vi "GetGrabberPosition.vi"(8 "error in (no error)":errorcluster, 11 "JKI.Robot.SMO":refnum<class "JKI.Robot.SMO.lvclass">) -> (0 "error out":errorcluster, 2 "SetGrabberPosition":dbl, 3 "JKI.Robot.SMO out":refnum<class "JKI.Robot.SMO.lvclass">)   [LabVIEW 2015, in "JKI.Robot.SMO.lvclass"]
doc: "---------------------------------------------------------------\nJKI State Machine Objects™\nhttp://jki.net/state-machine-objects/\nCopyright (C) 2005-2015, JKI <info@jki.net>\nALL RIGHTS RESERVEDJKI State Machine Objects (SMO) 1.0.0.4\nJKI - JKI\nCopyright (c) 2015, JKI"
uses:
  JKI.Robot.SMO.lvclass
  JKI.Robot.SMO.lvclass/JKI.Robot.SMO.ctl
panel:
  # "For instructions on how to use the JKI State Machine Objects, examples and video tutorials, visit:\nhttp://jki.net/state-machine-objects/\n\nJKI State Machine Objects™\nhttp://jki.net/state-machine-objects/\nCopyright (C) 2005-2015, JKI <info@jki.net>\nALL RIGHTS RESERVED"
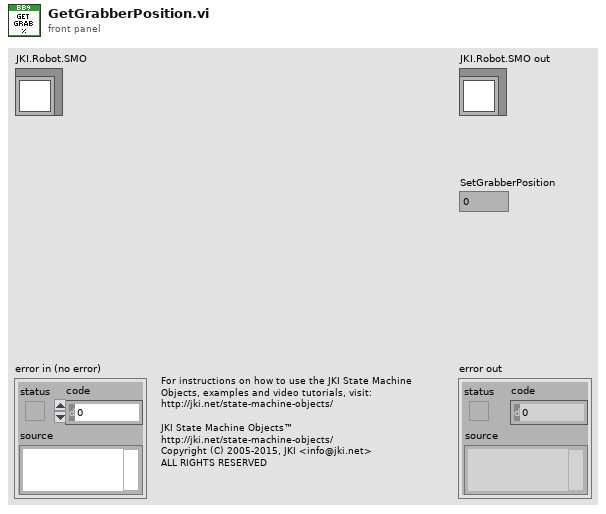
[diagram p1: front panel]
types:
  T1 = typedef "JKI.Robot.SMO.lvclass/PrivateData--Ref.ctl" = refnum<data-value>
  T2 = typedef "JKI.Robot.SMO.lvclass/PrivateData--Cluster.ctl" = cluster{"Configuration":T3, "Public Events":T4, "Robot Position":T5, "Private Events":T6}
  T3 = typedef "JKI.Robot.SMO.lvclass/Configuration--Cluster.ctl" = cluster{"Suffix":string}
  T4 = typedef "JKI.Robot.SMO.lvclass/PublicEvents--Cluster.ctl" = cluster{"Data Changed":refnum<user-event>}
  T5 = typedef "RobotPosition--Cluster.ctl" = cluster{"Claw":dbl, "JointA":dbl, "JointB":dbl, "JointC":dbl, "JointD":dbl}
  T6 = typedef "JKI.Robot.SMO.lvclass/PrivateEvents--Cluster.ctl" = cluster{"SetGrabberPosition":refnum<user-event>, "SetJointRotation":refnum<user-event>}
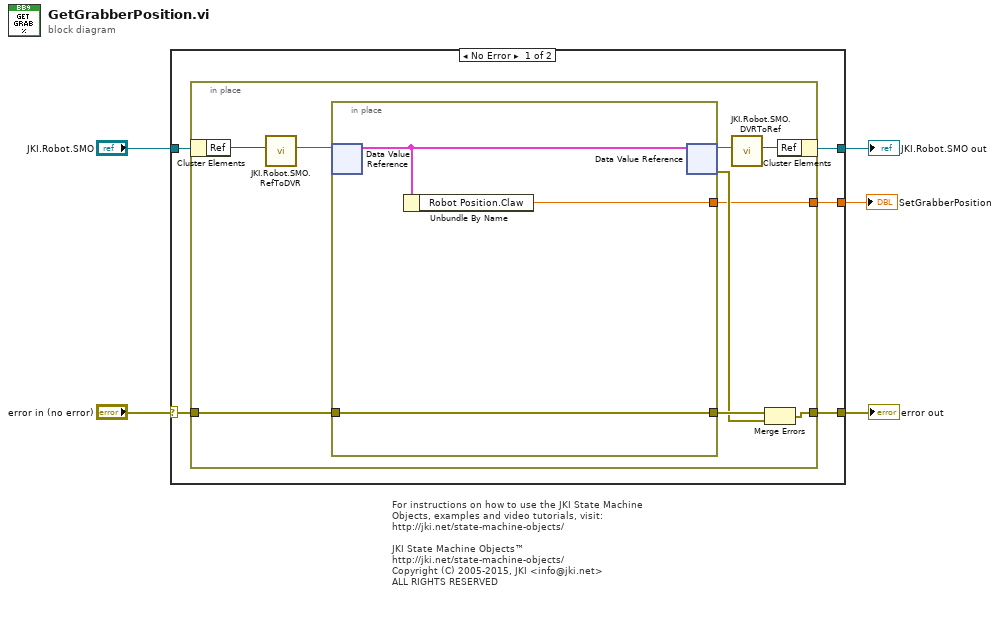
[diagram p0: block diagram]
diagram:
  # "For instructions on how to use the JKI State Machine Objects, examples and video tutorials, visit:\nhttp://jki.net/state-machine-objects/\n\nJKI State Machine Objects™\nhttp://jki.net/state-machine-objects/\nCopyright (C) 2005-2015, JKI <info@jki.net>\nALL RIGHTS RESERVED"
  n1 = case shown="No Error" "error in (no error)" {
    selector: "error in (no error)" -> [w8 w24]
    tunnel: [w7 w24] -> w4
    tunnel: [w9 w23] -> w5
    tunnel: "JKI.Robot.SMO" -> [w10 w23]
    tunnel: [w6 _] -> w1
    frame No Error {
      n2 = in-place {
        in-place-border: w8 -> [w19]
        in-place-border: [w16] -> w7
        in-place-border: [w11] -> w6
        n3 = in-place-cluster #1(w10) -> ("Ref"=w15:u32)
        n4 = call "JKI.Robot.SMO.RefToDVR.vi"("Ref"=w15) -> ("Ref"=w13:T1)  [unwired: 10 in]
        n5 = in-place {
          in-place-border: w19 -> [w20]
          in-place-border: [w20] -> w18
          in-place-border: [w21] -> w11
          n6 = in-place-dvr #2(w13) -> (w22:T2)  [unwired: 1 out]
          n7 = Unbundle By Name(w22) -> ("Robot Position.Claw"=w21:dbl)
          n8 = in-place-dvr #2(w22) -> (w14:T1, w17:errorcluster)
        }
        n9 = call "JKI.Robot.SMO.DVRToRef.vi"("Ref"=w14) -> ("Ref"=w12:u32)  [unwired: 10 in]
        n10 = Merge Errors(w18, w17) -> (w16:errorcluster)
        n11 = in-place-cluster #1("Ref"=w12) -> (w9:refnum<class "JKI.Robot.SMO.lvclass">)
      }
    }
    frame Error {
    }
  }
  "error out" <- w4
  "JKI.Robot.SMO out" <- w5
  "SetGrabberPosition" <- w1
